vi "Get Position Piezo.vi"(5 "Piezo State":T2, 7 "Counter Time":i32, 8 "error in (no error)":errorcluster, 9 "notifier out":refnum<notifier>, 11 "Hardware Configuration":T1) -> (0 "error out":errorcluster, 1 "VOLTAGE":dbl(knob) scale=0.0..10.0, 2 "ACTUAL POSITION \n[MICRON]":dbl[](array[numeric]), 3 "Hardware Configuration 2":T1, 4 "x*y":dbl[](graph))   [LabVIEW 2013, in "Piezo.lvlib"]
uses:
  Piezo/Piezo.lvlib
  Hardware Configuration Piezo.ctl
  Piezo/Piezo State.ctl
  Piezo/Piezo display.ctl
  <vilib>/DAQmx/read.llb/DAQmx Read (Analog Wfm 1Chan NSamp).vi
panel:
  out "DAQmx Task":refnum<k21>
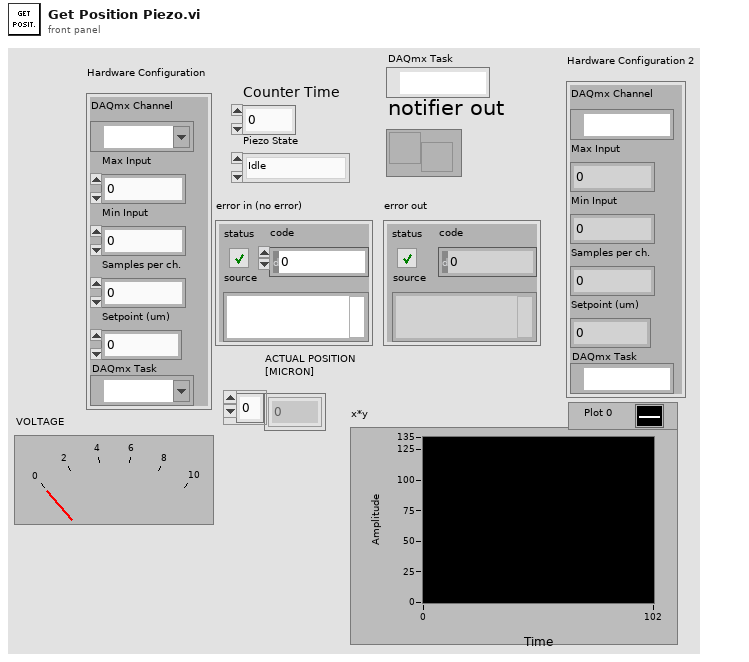
[diagram p1: front panel]
types:
  T1 = typedef "Piezo.lvlib/Hardware Configuration Piezo.ctl" = cluster{"DAQmx Channel":tag, "Max Input":dbl, "Min Input":dbl, "Samples per ch.":dbl, "Setpoint (um)":dbl, "DAQmx Task":refnum<k21>}
  T2 = typedef "Piezo.lvlib/Piezo State.ctl" = enum16{"Idle", "Acquiring"}
  T3 = typedef "Piezo.lvlib/Piezo display.ctl" = cluster{"PiezoPosition":sgl, "Counter Time":i32}
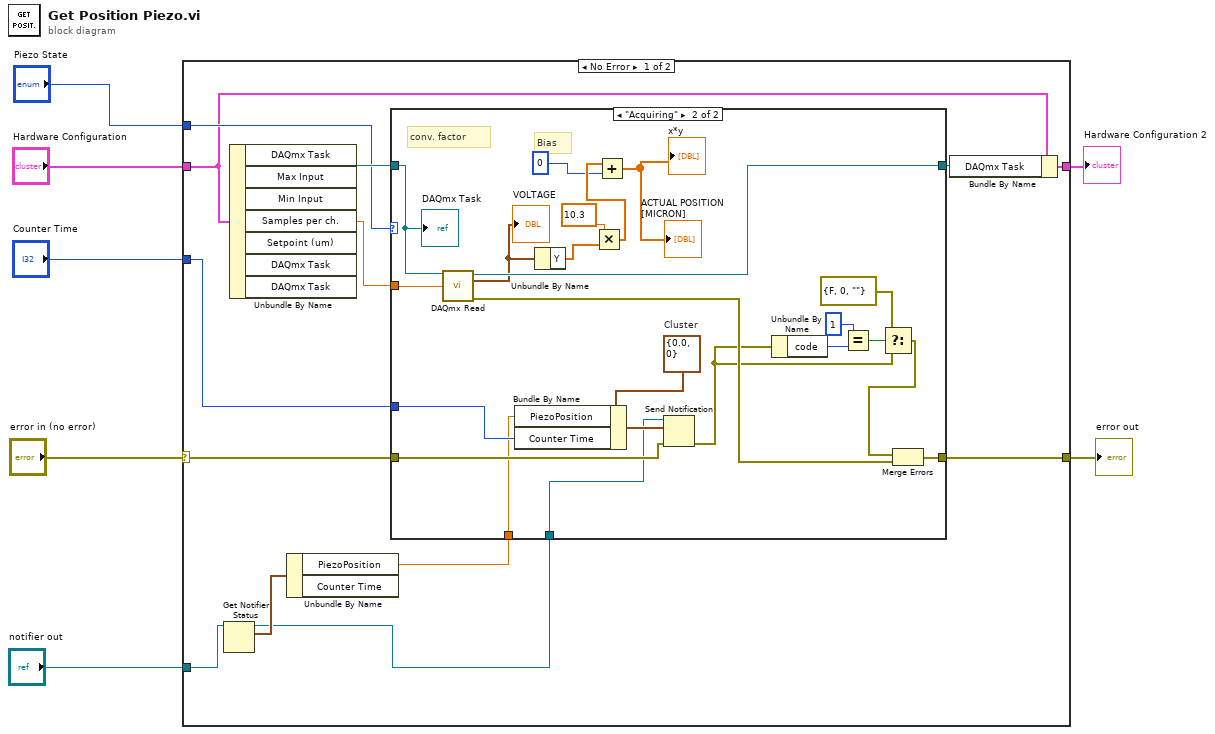
[diagram p0: block diagram]
diagram:
  n1 = case shown="No Error" "error in (no error)" {
    selector: "error in (no error)" -> [w14 w46]
    tunnel: [w13 w46] -> w6
    tunnel: "Hardware Configuration" -> [w16 w47]
    tunnel: "Piezo State" -> [w17 _]
    tunnel: [w18 w47] -> w3
    tunnel: "Counter Time" -> [w15 _]
    tunnel: "notifier out" -> [w10 _]
    frame No Error {
      n2 = Get Notifier Status(notifier=w10) -> (notifier out=w9:refnum<notifier>, current notification=w11:T3)  [unwired: 1 in, 3 out]
      n3 = Unbundle By Name(w16) -> ("DAQmx Task"=w20:refnum<k21>, "Samples per ch."=w12:dbl)  [unwired: 5 out]
      n4 = Unbundle By Name(w11) -> ("PiezoPosition"=w8:sgl)  [unwired: 1 out]
      n5 = case shown="\"Acquiring\"" w17 {
        tunnel: w20 -> [w22 w40]
        tunnel: [w22 w39] -> w19
        tunnel: w15 -> [_ w42]
        tunnel: w9 -> [_ w31]
        tunnel: w14 -> [w21 w43]
        tunnel: [w21 w44] -> w13
        tunnel: w12 -> [_ w37]
        tunnel: w8 -> [_ w23]
        frame "Idle", Default {
        }
        frame "Acquiring" {
          w41 = T3 {"PiezoPosition"=0.0, "Counter Time"=0}  # Cluster
          # "conv. factor"
          # "Bias"
          n6 = call-poly <vilib>:"DAQmx Read.vi"("task/channels in"=w40, "number of samples per channel"=w37) -> ("task out"=w39:refnum<k21>, "data"=w30:waveform(dbl), "error out"=w38:errorcluster)  [unwired: 11 in]
          "VOLTAGE" <- w30
          n7 = Bundle By Name(cluster=w41, "PiezoPosition"=w23, "Counter Time"=w42) -> (w45:T3)
          n8 = Unbundle By Name(w30) -> ("Y"=w27:dbl[])
          n9 = Multiply(x=10.3, y=w27) -> (x*y=w25:dbl[])
          n10 = Add(x=w25, y=0) -> (x+y=→"ACTUAL POSITION \n[MICRON]" →"x*y":dbl[])
          n11 = Send Notification(notification=w45, notifier=w31, error in (no error)=w43) -> (error out=w29:errorcluster)  [unwired: 1 out]
          n12 = Unbundle By Name(w29) -> ("code"=w36:i32)
          n13 = Equal?(x=1, y=w36) -> (x = y?=w34:bool)
          n14 = Select(t=errorcluster {"status"=FALSE, "code"=0, "source"=""} ("error constant"), s=w34, f=w29) -> (s? t:f=w32:errorcluster)
          n15 = Merge Errors(w32, w38) -> (w44:errorcluster)
          "DAQmx Task" <- w40
        }
      }
      n16 = Bundle By Name(cluster=w16, "DAQmx Task"=w19) -> (w18:T1)
    }
    frame Error {
    }
  }
  "error out" <- w6
  "Hardware Configuration 2" <- w3
